vi "Init Runtime.vi"(8 "error in (no error)":errorcluster, 11 "Formatter Config in":refnum<class "Formatter Config.lvclass">) -> (0 "error out":errorcluster, 2 "Formatter.lvclass":refnum<class "Formatter.lvclass">, 3 "Formatter Config out":refnum<class "Formatter Config.lvclass">)   [LabVIEW 2015, in "Formatter Config.lvclass"]
uses:
  Formatter Config.lvclass
  Execution/Formatter.lvclass
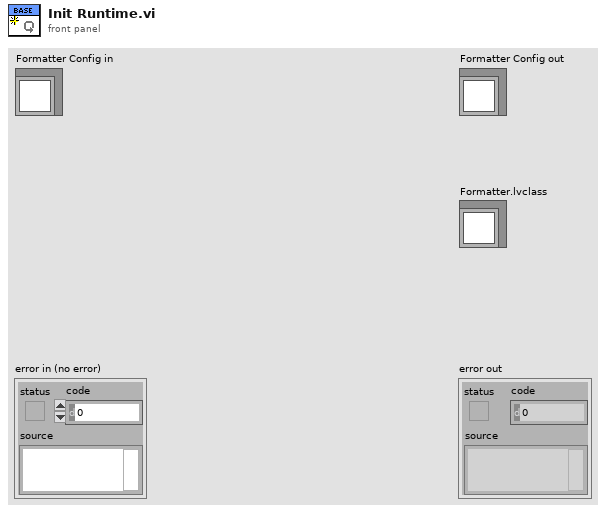
[diagram p1: front panel]
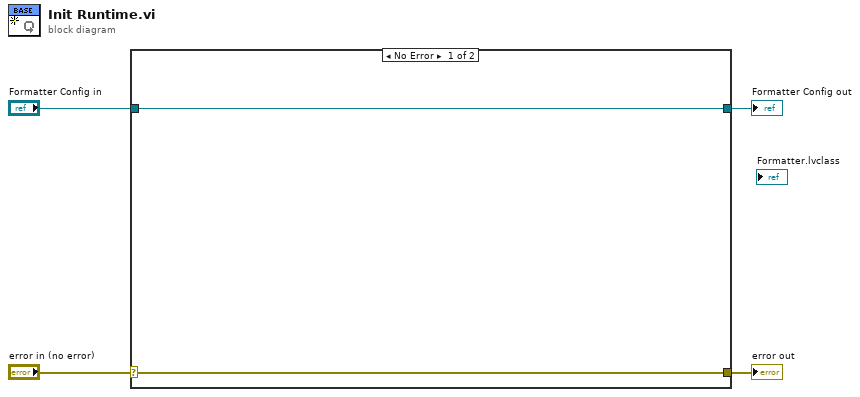
[diagram p0: block diagram]
diagram:
  n1 = case shown="No Error" "error in (no error)" {
    selector: "error in (no error)" -> [w5 w8]
    tunnel: [w5 w8] -> w3
    tunnel: [w6 w7] -> w1
    tunnel: "Formatter Config in" -> [w6 w7]
    frame No Error {
    }
    frame Error {
    }
  }
  "error out" <- w3
  "Formatter Config out" <- w1
